vi "Launch Channel Selection Dialog.vi"(8 "error in (no error)":errorcluster, 10 "Channels to Highlight":string[](array[string]), 11 "SDF Path":path) -> (0 "error out":errorcluster, 2 "Channels Selected":string[](array[string]), 3 "SysDef Path Out":path)   [LabVIEW 2015]
uses:
  NationalInstruments.VeriStand.SystemStorageUI
  NationalInstruments.VeriStand.SystemDefinitionAPI
  NationalInstruments.VeriStand.SystemStorage
panel:
  in  "Cancel":bool
  in  "OK":bool
  in  "TreeBrowserWF":refnum<k24>(container)
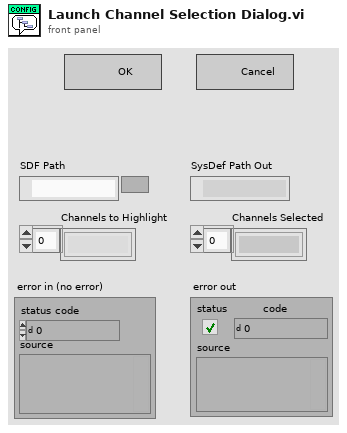
[diagram p1: front panel]
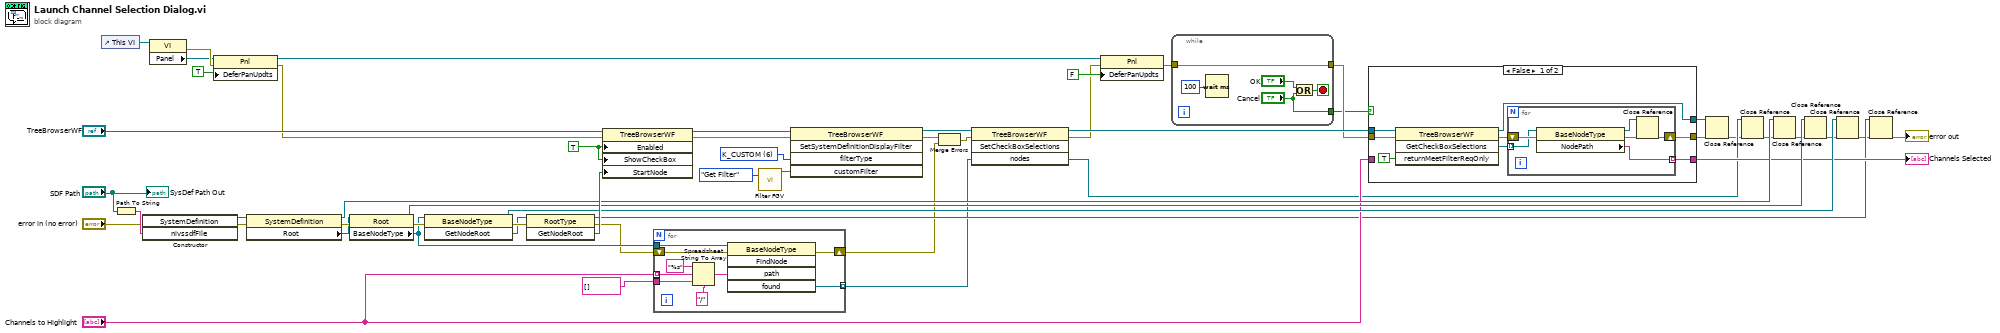
[diagram p0: block diagram]
diagram:
  w29 = u8 6 items=["K_CHAN_R", "K_CHAN_W", "K_CHAN_RW", "K_CHAN_VOLT", "K_CHAN_FAULT", "K_ALL", "K_CUSTOM", "K_CHAN_R_VIS", "K_CHAN_W_VIS", "K_CHAN_RW_VIS", "K_CHAN_VOLT_VIS", "K_CHAN_FAULT_VIS", "K_WAVE", "K_WAVE_VIS", "K_WAVE_DBL", "K_WAVE_CDB", "K_WAVE_DBL_VIS", "K_WAVE_CDB_VIS"] ("filterType")
  w52 = TRUE ("Enabled")
  n1 = control-ref of="This VI"() -> (w51:refnum<vi>)
  n2 = Path To String(path="SDF Path") -> (string=w46:string)
  n3 = constructor class="SystemDefinition"(error in="error in (no error)", "nivssdfFile"=w46) -> (reference out=w44:refnum<k24>, error out=w43:errorcluster)  [unwired: 2 in, 2 out]
  n4 = property class="VI"(reference=w51) -> (error out=w50:errorcluster, "Panel"=w49:refnum<vi>)  [unwired: 1 in, 1 out]
  n5 = property class="Pnl"(reference=w49, error in=w50, "DeferPanUpdts"=TRUE ("Defer Panel Updates")) -> (reference out=w47:refnum<vi>, error out=w39:errorcluster)
  n6 = property class="SystemDefinition"(reference=w44, error in=w43) -> (reference out=w33:refnum<k24>, error out=w42:errorcluster, "Root"=w41:refnum<k24>)
  n7 = property class="Root"(reference=w41, error in=w42) -> (reference out=w32:refnum<k24>, error out=w40:errorcluster, "BaseNodeType"=w25:refnum<k24>)
  n8 = invoke class="BaseNodeType" method="GetNodeRoot"(reference=w25, error in=w40) -> (reference out=w31:refnum<k24>, error out=w38:errorcluster, "GetNodeRoot"=w26:refnum<k24>)  [unwired: 1 in]
  n9 = invoke class="RootType" method="GetNodeRoot"(reference=w26, error in=w38) -> (reference out=w12:refnum<k24>, error out=w24:errorcluster, "GetNodeRoot"=w37:refnum<k24>)  [unwired: 1 in]
  n10 = property class="TreeBrowserWF"(reference="TreeBrowserWF", error in=w39, "Enabled"=w52, "ShowCheckBox"=w52, "StartNode"=w37) -> (reference out=w35:refnum<k24>, error out=w36:errorcluster)
  n11 = for {
    tunnel: w25 -> [w62]
    shift-right: [w60] -> w10
    shift-left: w24 -> [w61]
    tunnel: "Channels to Highlight" -> [w57] mode=indexing
    tunnel: string[] [] -> [w56]
    tunnel: [w54] -> w11 mode=indexing
    n12 = Spreadsheet String To Array(delimiter (Tab)="/", format string="%s", spreadsheet string=w57, array type (2D Dbl)=w56) -> (array=w55:string[])
    n13 = invoke class="BaseNodeType" method="FindNode"(reference=w62, error in=w61, "path"=w55) -> (error out=w60:errorcluster, "found"=w54:refnum<k24>)  [unwired: 2 in, 3 out]
  }
  n14 = call "Filter FGV.vi"("Enum"=enum16{"Get Filter", "Add GUIDs"}."Get Filter") -> ("Filter Out"=w2:refnum<k24>)  [unwired: 9 in, 1 out]
  n15 = invoke class="TreeBrowserWF" method="SetSystemDefinitionDisplayFilter"(reference=w35, error in=w36, "filterType"=w29, "customFilter"=w2) -> (reference out=w28:refnum<k24>, error out=w34:errorcluster)  [unwired: 1 in, 3 out]
  n16 = Merge Errors(w34, w10) -> (w21:errorcluster)
  n17 = invoke class="TreeBrowserWF" method="SetCheckBoxSelections"(reference=w28, error in=w21, "nodes"=w11) -> (reference out=w27:refnum<k24>, error out=w9:errorcluster, "nodes"=w13:refnum<k24>[])  [unwired: 1 in, 1 out]
  n18 = property class="Pnl"(reference=w47, error in=w9, "DeferPanUpdts"=FALSE ("Defer Panel Updates")) -> (error out=w8:errorcluster)  [unwired: 1 out]
  n19 = while {
    tunnel: w8 -> [w66]
    tunnel: [w66] -> w20
    tunnel: ["Cancel"] -> w16
    stop <- w65 stop-if-true
    n20 = Wait (ms)(milliseconds to wait=u32 100) -> ()  [unwired: 1 out]
    n21 = Or(x="OK", y="Cancel") -> (x .or. y?=w65:bool)
  }
  n22 = case shown="False" w16 {
    tunnel: w27 -> [w75 w84]
    tunnel: w20 -> [w74 w82]
    tunnel: [w71 w82] -> w19
    tunnel: [w70 w84] -> w18
    tunnel: [w68 w83] -> w17
    tunnel: "Channels to Highlight" -> [_ w83]
    frame False {
      n23 = invoke class="TreeBrowserWF" method="GetCheckBoxSelections"(reference=w75, error in=w74, "returnMeetFilterReqOnly"=TRUE) -> (reference out=w70:refnum<k24>, error out=w72:errorcluster, "GetCheckBoxSelections"=w73:refnum<k24>[])  [unwired: 1 in, 1 out]
      n24 = for {
        tunnel: w73 -> [w80] mode=indexing
        shift-right: [w78] -> w71
        shift-left: w72 -> [w81]
        tunnel: [w76] -> w68 mode=indexing
        n25 = property class="BaseNodeType"(reference=w80, error in=w81) -> (reference out=w77:refnum<k24>, error out=w79:errorcluster, "NodePath"=w76:string)
        n26 = Close Reference(reference=w77, error in (no error)=w79) -> (error out=w78:errorcluster)
      }
    }
    frame True {
    }
  }
  "Channels Selected" <- w17
  n27 = Close Reference(reference=w18, error in (no error)=w19) -> (error out=w7:errorcluster)
  n28 = Close Reference(reference=w13, error in (no error)=w7) -> (error out=w5:errorcluster)
  n29 = Close Reference(reference=w33, error in (no error)=w5) -> (error out=w6:errorcluster)
  n30 = Close Reference(reference=w32, error in (no error)=w6) -> (error out=w4:errorcluster)
  n31 = Close Reference(reference=w31, error in (no error)=w4) -> (error out=w3:errorcluster)
  n32 = Close Reference(reference=w12, error in (no error)=w3) -> (error out=→"error out":errorcluster)
  "SysDef Path Out" <- "SDF Path"
